vi "XTrend_Facade.vi"(0 "Data In":T5, 2 "Display State In":T2, 3 "Container State":T4) -> (6 "Data Out":T5, 7 "Display State Out":T2, 8 "Action":T1)   [LabVIEW 2015, in "XTrend.xctl"]
uses:
  XTrend.xctl
  XTrend_Data.ctl
  <vilib>/_xctls/Container State.ctl
  XTrend_State.ctl
  View Mode.ctl
  <vilib>/_xctls/Action.ctl
  <vilib>/_xctls/XControlSupport.lvlib
panel:
  out "System Waveform Graph":dbl[](graph) caption="Raw Data"
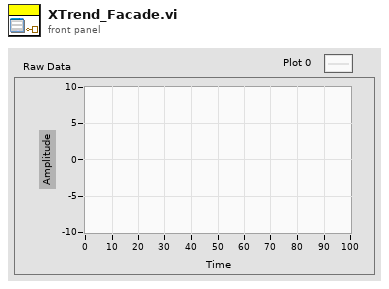
[diagram p1: front panel]
types:
  T1 = typedef "XControlSupport.lvlib/Action.ctl" = cluster{"Data Changed?":bool, "State Changed?":bool, "Action Name":string}
  T2 = typedef "XTrend.xctl/XTrend_State.ctl" = cluster{"View Mode":T3, "Trend Count":dbl}
  T3 = typedef "View Mode.ctl" = enum16{"Raw Data", "Trend"}
  T4 = typedef "XControlSupport.lvlib/Container State.ctl" = cluster{"Indicator?":bool, "Run Mode?":bool, " Refnum":refnum<vi>}
  T5 = typedef "XTrend.xctl/XTrend_Data.ctl" = dbl[]
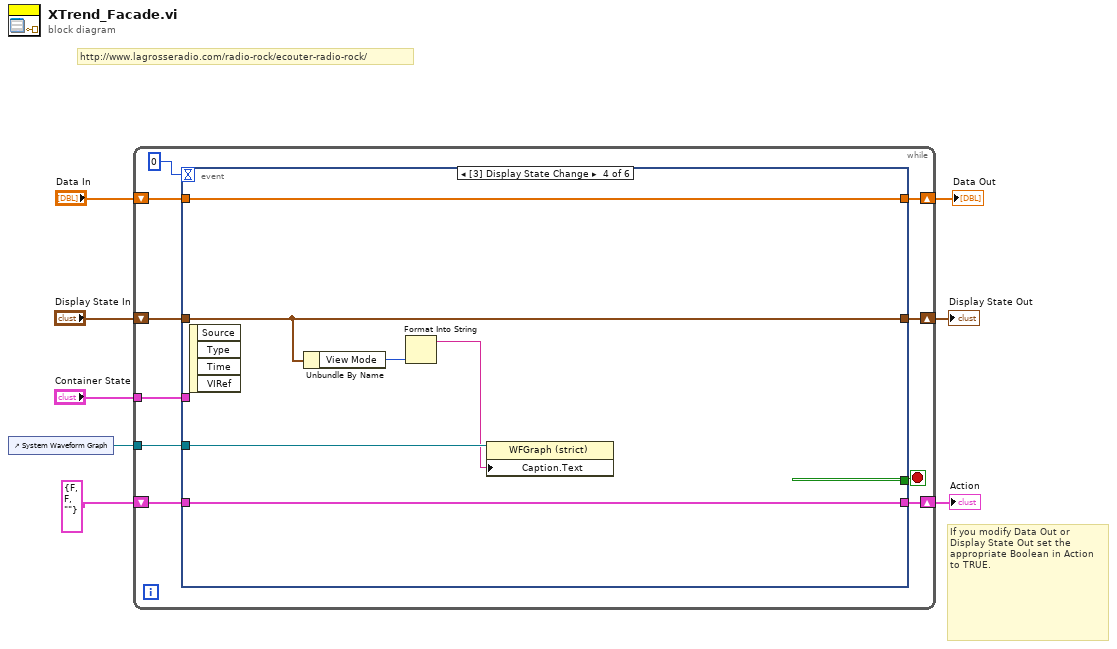
[diagram p0: block diagram]
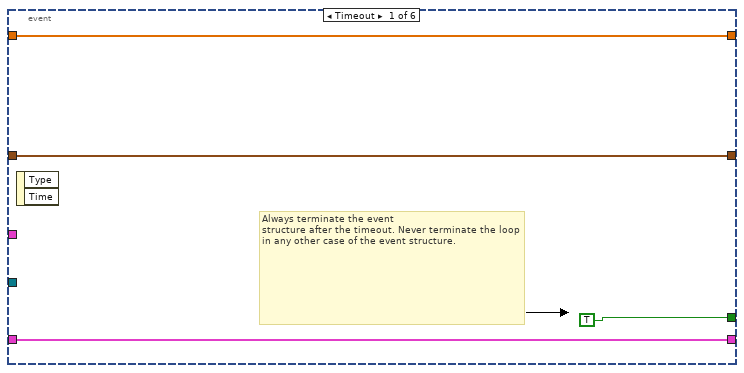
[diagram p2: hidden frame]
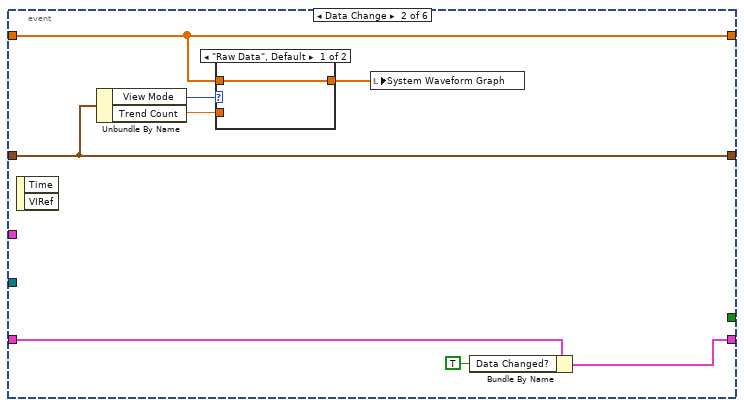
[diagram p3: hidden frame]
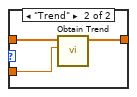
[diagram p4: hidden frame]
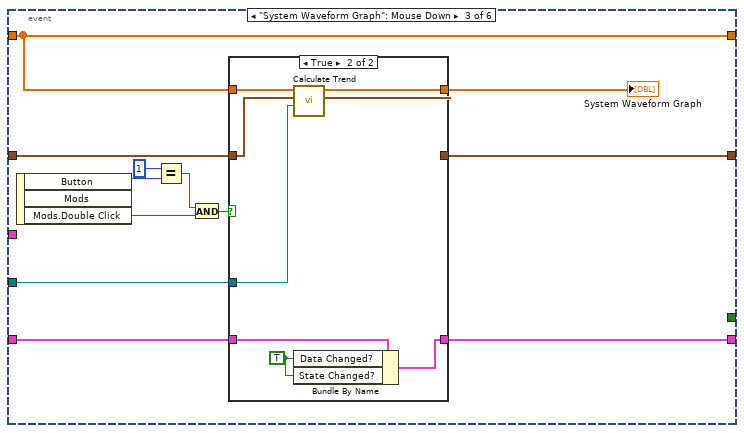
[diagram p5: hidden frame]
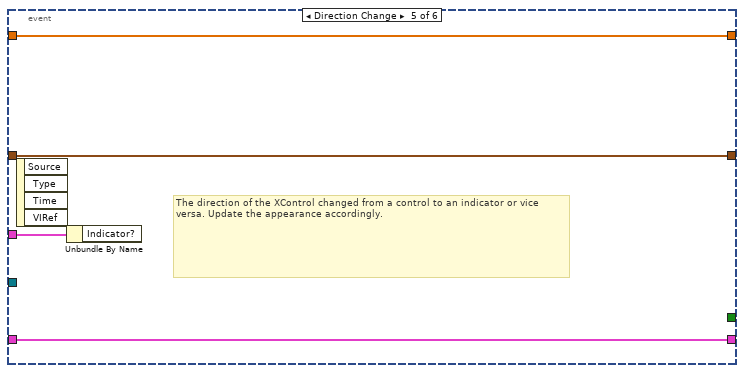
[diagram p7: hidden frame]
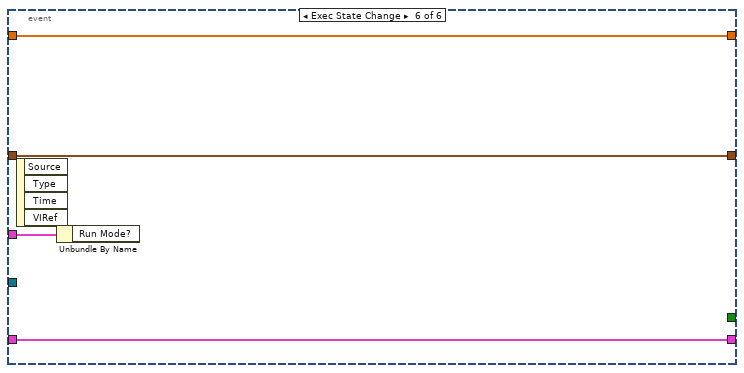
[diagram p8: hidden frame]
diagram:
  # "http://www.lagrosseradio.com/radio-rock/ecouter-radio-rock/"
  # "If you modify Data Out or\nDisplay State Out set the\nappropriate Boolean in Action\nto TRUE."
  n1 = control-ref of="System Waveform Graph"() -> (w1:refnum<vi>)
  n2 = while {
    shift-right: [w17] -> w7
    shift-left: "Display State In" -> [w18]
    tunnel: "Container State" -> [w14]
    shift-right: [w12] -> w5
    shift-left: T1 {"Data Changed?"=FALSE, "State Changed?"=FALSE, "Action Name"=""} ("Action") -> [w13]
    shift-right: [w10] -> w2
    shift-left: "Data In" -> [w11]
    tunnel: w1 -> [w9]
    stop <- w16 stop-if-true
    n3 = event shown="[3] Display State Change" {
      selector: _ -> [_ _ _ _ _ _]
      dyn-events: _ -> [_ _ _ _ _ _]
      timeout: 0 -> [_ _ _ _ _ _]
      tunnel: w18 -> [w20 w29 w42 w61 w66 w70]
      tunnel: [w20 w29 w41 w61 w66 w70] -> w17
      tunnel: [TRUE _ _ _ _ _] -> w16
      tunnel: w14 -> [_ _ _ _ w67 w71]
      tunnel: [w21 w28 w38 w63 w65 w69] -> w12
      tunnel: w13 -> [w21 w30 w39 w63 w65 w69]
      tunnel: w11 -> [w19 w24 w37 w62 w64 w68]
      tunnel: [w19 w24 w37 w62 w64 w68] -> w10
      tunnel: w9 -> [_ _ w35 w59 _ _]
      event Timeout {
        # "Always terminate the event\nstructure after the timeout. Never terminate the loop in any other case of the event structure."
        n4 = event-data() -> ()  [unwired: 1 in, 2 out]
      }
      event Data Change {
        n5 = event-data() -> ()  [unwired: 1 in, 2 out]
        n6 = Unbundle By Name(w29) -> ("View Mode"=w26:T3, "Trend Count"=w25:dbl)
        n7 = case shown="\"Raw Data\", Default" w26 {
          tunnel: [w31 w33] -> w23
          tunnel: w25 -> [_ w34]
          tunnel: w24 -> [w31 w32]
          frame "Raw Data", Default {
          }
          frame "Trend" {
            n8 = call "Obtain Trend.vi"("Trend Count"=w34, "Data In"=w32) -> ("Array"=w33:dbl[])  [unwired: 9 in]
          }
        }
        n9 = local write "System Waveform Graph"(w23) -> ()
        n10 = Bundle By Name(cluster=w30, "Data Changed?"=TRUE) -> (w28:T1)
      }
      event "System Waveform Graph": Mouse Down {
        n11 = event-data() -> ("Button"=w46:u16, "Mods.Double Click"=w44:bool)  [unwired: 1 in, 1 out]
        n12 = Equal?(x=u16 1, y=w46) -> (x = y?=w43:bool)
        n13 = And(x=w43, y=w44) -> (x .and. y?=w40:bool)
        n14 = case shown="True" w40 {
          tunnel: w42 -> [w49 w51]
          tunnel: [w49 w57] -> w41
          tunnel: [w47 w56] -> w36
          tunnel: w39 -> [w48 w54]
          tunnel: [w48 w53] -> w38
          tunnel: w37 -> [w47 w52]
          tunnel: w35 -> [_ w50]
          frame False {
          }
          frame True {
            w55 = TRUE ("Data Changed?")
            n15 = call "Calculate Trend.vi"("WaveformGraph in"=w50, "Display State In in"=w51, "Data In in"=w52) -> ("Display State In out"=w57:T2, "Data In out"=w56:T5)  [unwired: 7 in]
            n16 = Bundle By Name(cluster=w54, "Data Changed?"=w55, "State Changed?"=w55) -> (w53:T1)
          }
        }
        "System Waveform Graph" <- w36
      }
      event Display State Change {
        n17 = event-data() -> ()  [unwired: 1 in, 4 out]
        n18 = Unbundle By Name(w61) -> ("View Mode"=w60:T3)
        n19 = Format Into String(w60) -> (resulting string=w58:string)  [unwired: 3 in, 1 out]
        n20 = property class="WFGraph (strict)"(reference=w59, "Caption.Text"=w58) -> ()  [unwired: 1 in, 2 out]
      }
      event Direction Change {
        # "The direction of the XControl changed from a control to an indicator or vice versa. Update the appearance accordingly."
        n21 = event-data() -> ()  [unwired: 1 in, 4 out]
        n22 = Unbundle By Name(w67) -> ()  [unwired: 1 out]
      }
      event Exec State Change {
        n23 = event-data() -> ()  [unwired: 1 in, 4 out]
        n24 = Unbundle By Name(w71) -> ()  [unwired: 1 out]
      }
    }
  }
  "Display State Out" <- w7
  "Data Out" <- w2
  "Action" <- w5
